vi "RSZVB Set Source Power Calibration Converter State.vi"(7 "Calibration Converter (On)":bool=TRUE, 8 "error in (no error)":errorcluster {"code" format="%.0x"}, 9 "Converter (1)":i32=1, 10 "Channel (1)":i32=1, 11 "VISA session":refnum<visa-resource-name>) -> (0 "error out":errorcluster {"code" format="%.0x"}, 3 "dup VISA session":refnum<visa-resource-name>)   [LabVIEW 2011]
doc: "This VI enables or disables the source power calibration for channel <Ch> and for an external frequency converter number <Con>. The converter must be equipped with an electronic attenuator (R&S ZVAZxxxE).\nThe command is disabled unless a source power calibration for the external converter has been performed (SOURce<Ch>:POWer<Pt>:CORRection[:ACQuire] CONVerter,\n<source_pt>). To enable or disable a source power calibration for an analyzer port use SOURce<Ch>:POWer<Pt>:CORRection[:STATe].\n\nRemote-control command(s):\nSOURce<Ch>:POWer<Pt>:CORRection:CONVerter<Con>[:STATe] <Boolean>"
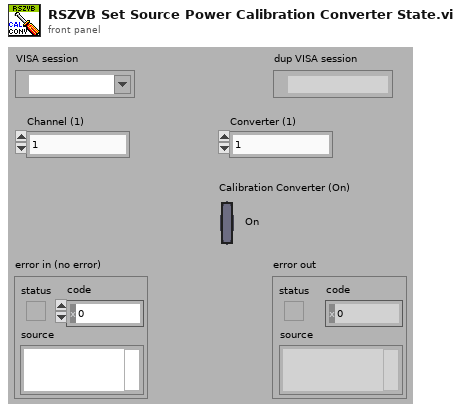
[diagram p1: front panel]
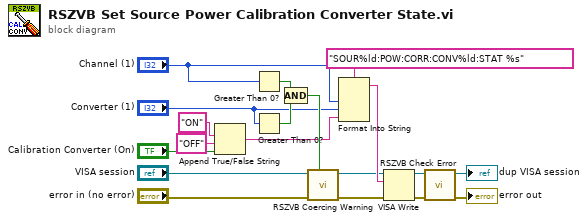
[diagram p0: block diagram]
diagram:
  n1 = Append True/False String(1:"Calibration Converter (On)", 2:"OFF" ("false string"), 3:"ON" ("true string")) -> (0:w8:string)  [unwired: 1 in]
  n2 = Greater Than 0?(x="Channel (1)") -> (x > 0?=w11:bool)
  n3 = Greater Than 0?(x="Converter (1)") -> (x > 0?=w10:bool)
  n4 = Compound Arithmetic op=AND(w11, w10) -> (w9:bool)
  n5 = call "RSZVB Coercing Warning.vi"("In Range?"=w9, "error in (no error)"="error in (no error)", "VISA session"="VISA session") -> ("error out"=w16:errorcluster, "dup VISA session"=w15:refnum<visa-resource-name>)  [unwired: 7 in]
  n6 = Format Into String(format string="SOUR%ld:POW:CORR:CONV%ld:STAT %s", "Channel (1)", "Converter (1)", w8) -> (resulting string=w19:string)  [unwired: 2 in, 1 out]
  n7 = VISA Write(VISA resource name=w15, write buffer=w19, error in (no error)=w16) -> (VISA resource name out=w18:refnum<visa-resource-name>, error out=w17:errorcluster)  [unwired: 1 out]
  n8 = call "RSZVB Check Error.vi"("error in (no error)"=w17, "VISA session"=w18) -> ("error out"=→"error out":errorcluster, "dup VISA session"=→"dup VISA session":refnum<visa-resource-name>)  [unwired: 8 in]
